vi "VIToVariant.vi"(1 "Prefix":string, 2 "VI Reference":refnum<vi>) -> (0 "VI Variant":variant)   [LabVIEW 2014]
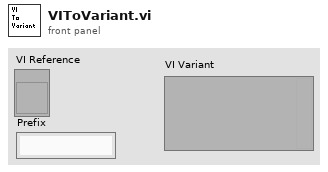
[diagram p1: front panel]
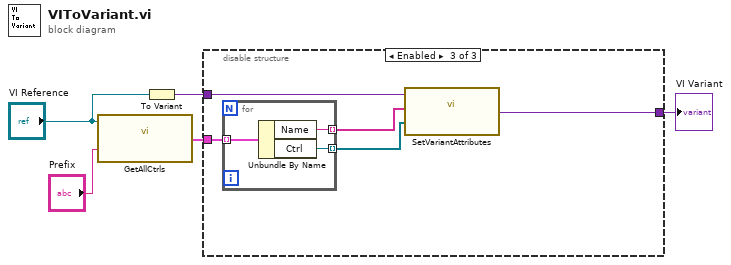
[diagram p0: block diagram]
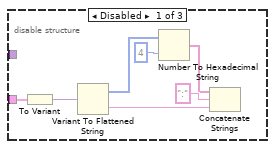
[diagram p2: hidden frame]
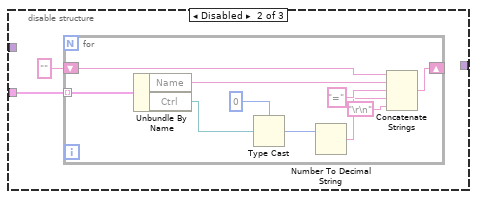
[diagram p3: hidden frame]
diagram:
  n1 = call "GetAllCtrls.vi"("Prefix"="Prefix", "VI"="VI Reference") -> ("Ctrls"=w2:cluster{"Name":string, "Ctrl":refnum<vi>}[])
  n2 = To Variant(anything="VI Reference") -> (Variant=w5:variant)
  n3 = disable-structure shown="Enabled" {
    disable-tunnel: w2 -> [w6 w13 w26]
    disable-tunnel: w5 -> [_ _ w27]
    disable-tunnel: [_ _ w25] -> w1
    frame Disabled {
      n4 = To Variant(anything=w6) -> (Variant=w8:variant)
      n5 = Variant To Flattened String(Variant=w8) -> (data string=w9:string, 1:w12:i16[])
      n6 = Number To Hexadecimal String(1:i16 4 ("width (-)"), 2:w12) -> (0:w10:string[])
      n7 = Concatenate Strings(w10, ":" ("data string"), w9) -> ()  [unwired: 1 out]
    }
    frame Disabled {
      n8 = for {
        tunnel: w13 -> [w24] mode=indexing
        shift-right: [w23] -> _
        shift-left: "" -> [w22]
        n9 = Unbundle By Name(w24) -> ("Name"=w21:string, "Ctrl"=w17:refnum<vi>)
        n10 = Type Cast(type=u32 0, x=w17) -> (*(type *) &x=w15:u32)
        n11 = Number To Decimal String(number=w15) -> (decimal integer string=w18:string)  [unwired: 1 in]
        n12 = Concatenate Strings(w22, w21, "=" ("string"), w18, "\r\n") -> (w23:string)
      }
    }
    frame Enabled {
      n13 = for {
        tunnel: w26 -> [w32] mode=indexing
        tunnel: [w31] -> w28 mode=indexing
        tunnel: [w30] -> w29 mode=indexing
        n14 = Unbundle By Name(w32) -> ("Name"=w31:string, "Ctrl"=w30:refnum<vi>)
      }
      n15 = call "SetVariantAttributes.vi"("values"=w29, "names"=w28, "Variant In"=w27) -> ("Variant Out"=w25:variant)
    }
  }
  "VI Variant" <- w1
